vi "SENSOR LM35-1.vi"() -> ()   [LabVIEW 2020]
uses:
  <vilib>/MakerHub/LINX/Public/Peripherals/Analog/Analog Read 1 Chan.vi
  <vilib>/MakerHub/LINX/Public/Peripherals/Digital/Digital Write 1 Chan.vi
  <vilib>/MakerHub/LINX/Public/Peripherals/Analog/Analog Read N Chans.vi
  <vilib>/MakerHub/LINX/Public/Peripherals/Digital/Digital Write N Chans.vi
  <vilib>/MakerHub/LINX/Private/Local IO/LinxAnalogRead.vi
  <vilib>/MakerHub/LINX/Public/Utilities/Check Channel.vi
  <vilib>/MakerHub/LINX/Private/Local IO/LinxDigitalWrite.vi
  <vilib>/MakerHub/LINX/Public/Utilities/Open Serial.vi
  <vilib>/MakerHub/LINX/Private/Utilties/Generate Error.vi
  <vilib>/MakerHub/LINX/LMH-LINX.lvlib
panel:
  out "> 60 C":bool
  out "35 - 60 C":bool
  out "FAHRENHEIT":dbl(knob) scale=0.0..212.0
  out "REAMUR":dbl(knob) scale=0.0..80.0
  out "KELVIN":dbl(knob) scale=273.0..373.0
  out "< 35 C":bool
  out "Grafik Suhu dengan LM35":dbl(graph)
  in  "Serial Port":refnum<visa-resource-name>="N/A"
  out "SUHU":dbl(knob) scale=0.0..100.0
  in  "?":bool
  # "PENGUKUR JARAK -  SENSOR SUHU LM35"
  # "Nama:\n1. Aldisya Putra Mahardika\n2. Aurelia Putri Widiyanta  \n3. Fahmi Fathur Rohman"
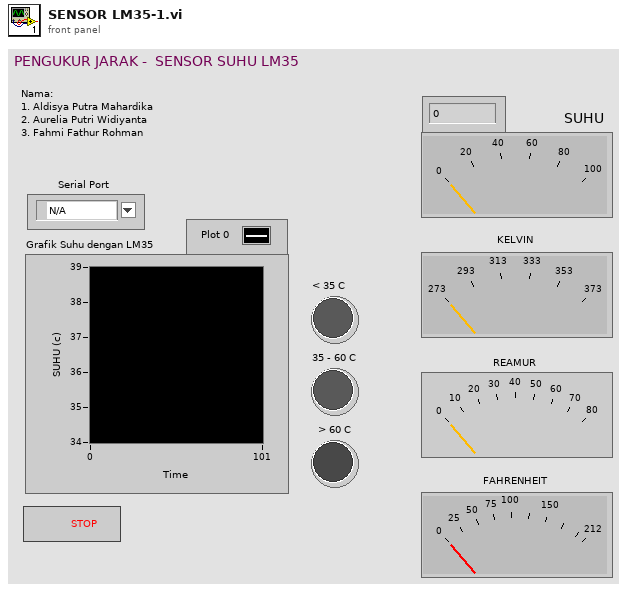
[diagram p1: front panel]
types:
  T1 = typedef "LMH-LINX.lvlib/LINX Ref.ctl" = cluster{"IO":T2, "Interface":T3, "LINX Device Config":T4}
  T2 = typedef "LMH-LINX.lvlib/Platform.ctl" = enum16{"Remote", "Local"}
  T3 = typedef "LMH-LINX.lvlib/Interface.ctl" = enum16{"Serial", "TCP"}
  T4 = typedef "LMH-LINX.lvlib/Device.lvlib/LINX Device Config.ctl" = cluster{"Interface":T3, "COM Port":refnum<visa-resource-name>, "TCP Configuration":T5, "Device Family":u8, "Device ID":u8, "Device Name":string, "TCP Ref":refnum<k5>, "Channels":T6}
  T5 = typedef "LMH-LINX.lvlib/Device.lvlib/TCP Config.ctl" = cluster{"IP Address":string, "Port":u16}
  T6 = typedef "LMH-LINX.lvlib/Channels.ctl" = cluster{"DI":u8[], "DO":u8[], "AI":u8[], "AO":u8[], "PWM":u8[], "QE":u8[], "UART":u8[], "I2C 2":u8[], "SPI":u8[], "CAN":u8[], "Servo":u8[], "AI Ref (V)":dbl, "AI Resolution (Bits)":u8, "AO Ref (V)":dbl, "AO Resolution (Bits)":u8}
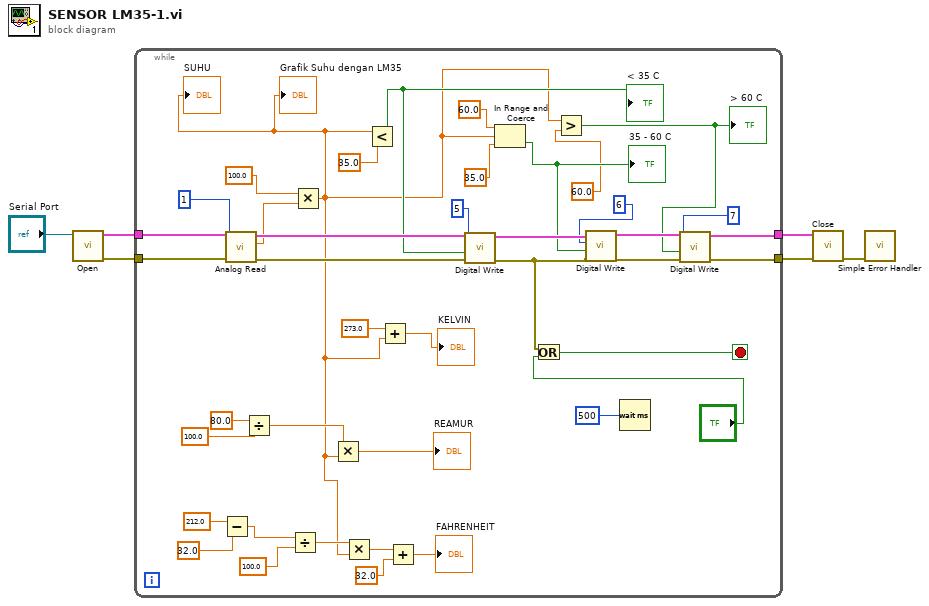
[diagram p0: block diagram]
diagram:
  n1 = call-poly <vilib>:"Open.vi"("Serial Port"="Serial Port") -> ("Error Out"=w4:errorcluster, "LINX Resource"=w6:T1)  [unwired: 8 in, 1 out]
  n2 = while {
    tunnel: w6 -> [w42]
    tunnel: [w34] -> w5
    tunnel: w4 -> [w44]
    tunnel: [w33] -> w3
    stop <- w45 stop-if-true
    n3 = Subtract(x=212.0, y=32.0) -> (x-y=w20:dbl)
    n4 = call-poly <vilib>:"Analog Read.vi"("Error In"=w44, "Analog Channel"=u8 1, "LINX Resource"=w42) -> ("Error Out"=w43:errorcluster, "Voltage"=w40:dbl, "LINX Resource"=w41:T1)  [unwired: 5 in, 1 out]
    n5 = Divide(x=80.0, y=100.0) -> (x/y=w24:dbl)
    n6 = Divide(x=w20, y=100.0) -> (x/y=w18:dbl)
    n7 = Multiply(x=100.0, y=w40) -> (x*y=w9:dbl)
    "SUHU" <- w9
    "Grafik Suhu dengan LM35" <- w9
    n8 = Multiply(x=w24, y=w9) -> (x*y=→"REAMUR":dbl)
    n9 = Multiply(x=w18, y=w9) -> (x*y=w17:dbl)
    n10 = Less?(x=w9, y=35.0) -> (x < y?=w13:bool)
    "< 35 C" <- w13
    n11 = Add(x=273.0, y=w9) -> (x+y=→"KELVIN":dbl)
    n12 = Add(x=w17, y=32.0) -> (x+y=→"FAHRENHEIT":dbl)
    n13 = call-poly <vilib>:"Digital Write.vi"("Error In"=w43, "Output Value"=w13, "DO Channel"=u8 5, "LINX Resource"=w41) -> ("Error Out"=w31:errorcluster, "LINX Resource"=w36:T1)  [unwired: 6 in]
    n14 = In Range and Coerce(upper limit=60.0, x=w9, lower limit=35.0) -> (In Range?=w10:bool)  [unwired: 1 out]
    "35 - 60 C" <- w10
    n15 = Or(x=w31, y="?") -> (x .or. y?=w45:bool)
    n16 = Greater?(x=w9, y=60.0) -> (0:w7:bool)
    "> 60 C" <- w7
    n17 = call-poly <vilib>:"Digital Write.vi"("Error In"=w31, "Output Value"=w10, "DO Channel"=u8 6, "LINX Resource"=w36) -> ("Error Out"=w32:errorcluster, "LINX Resource"=w35:T1)  [unwired: 6 in]
    n18 = Wait (ms)(milliseconds to wait=u32 500) -> ()  [unwired: 1 out]
    n19 = call-poly <vilib>:"Digital Write.vi"("Error In"=w32, "Output Value"=w7, "DO Channel"=u8 7, "LINX Resource"=w35) -> ("Error Out"=w33:errorcluster, "LINX Resource"=w34:T1)  [unwired: 6 in]
  }
  n20 = call <vilib>:"Close.vi"("Error In"=w3, "LINX Resource"=w5) -> ("Error Out"=w1:errorcluster)  [unwired: 9 in]
  n21 = call <vilib>:"Simple Error Handler.vi"("error in (no error)"=w1) -> ()  [unwired: 4 in, 5 out]
